vi "Program18.vi"() -> ()   [LabVIEW 2020]
panel:
  in  "Array 2":dbl[][](array[numeric])
  in  "Array":dbl[](array[numeric])
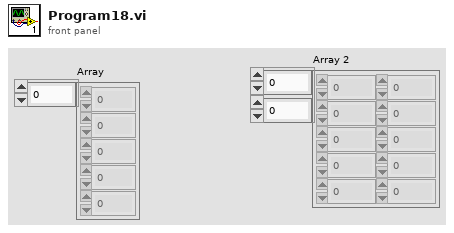
[diagram p1: front panel]
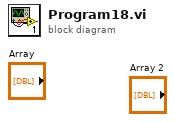
[diagram p0: block diagram]
diagram:
